vi "Trigger-time.vi"(8 "error in (no error)":errorcluster, 11 "Previous time":timestamp) -> (3 "Trigger time":timestamp)   [LabVIEW 2013, in "CameraVision.lvlib" / "CV-Acquisition.lvclass"]
uses:
  CV-Acquisition.lvclass
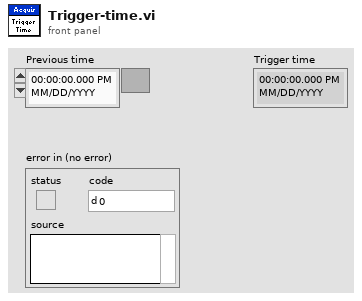
[diagram p1: front panel]
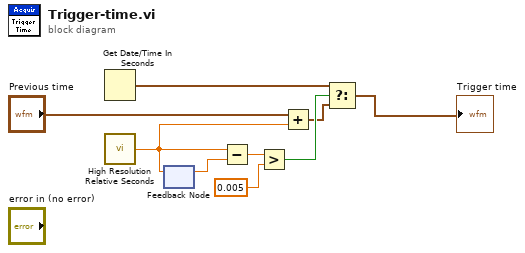
[diagram p0: block diagram]
diagram:
  n1 = Get Date/Time In Seconds() -> (seconds since 1Jan1904=w6:timestamp)
  n2 = call <vilib>:"High Resolution Relative Seconds.vi"() -> ("relative seconds"=w3:dbl)
  n3 = feedback-in #1(w3) -> ()
  n4 = feedback #1() -> (w4:dbl)  [unwired: 1 in]
  n5 = Subtract(x=w3, y=w4) -> (x-y=w9:dbl)
  n6 = Greater?(x=w9, y=0.005) -> (0:w7:bool)
  n7 = Add(x="Previous time", y=w3) -> (x+y=w1:timestamp)
  n8 = Select(t=w6, s=w7, f=w1) -> (s? t:f=→"Trigger time":timestamp)
